vi "Get Test Configuration Properties.vi"(8 "error in (no error)":errorcluster, 11 "Routing and Faulting System Tests in":refnum<class "Routing and Faulting System Tests.lvclass">) -> (0 "error out":errorcluster, 3 "Routing and Faulting System Tests out":refnum<class "Routing and Faulting System Tests.lvclass">)   [LabVIEW 2017, in "Routing and Faulting System Tests.lvclass"]
uses:
  Routing and Faulting System Tests.lvclass
  C:/dev/CustomDevice/niveristand-custom-device-testing-tools/VeriStandTestCase/VeriStandTestCase.lvclass
  Routing and Faulting System Tests.lvclass/Routing and Faulting System Tests.ctl
  niveristand-custom-device-testing-tools/VeriStandTestCase/VeriStandTestCase.lvclass
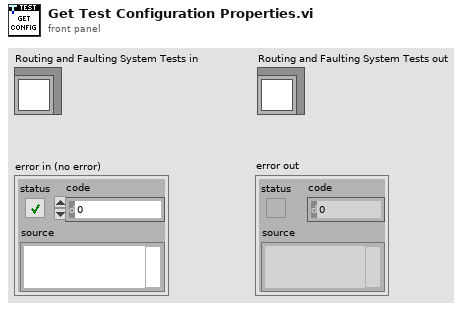
[diagram p1: front panel]
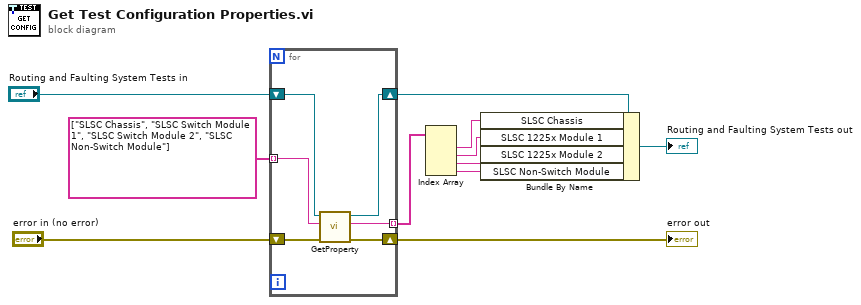
[diagram p0: block diagram]
diagram:
  n1 = for {
    tunnel: [w16] -> w6 mode=indexing
    shift-right: [w13] -> w3
    shift-left: "error in (no error)" -> [w15]
    tunnel: string[] ["SLSC Chassis", "SLSC Switch Module 1", "SLSC Switch Module 2", "SLSC Non-Switch Module"] -> [w14] mode=indexing
    shift-right: [w12] -> w1
    shift-left: "Routing and Faulting System Tests in" -> [w17]
    n2 = call "GetProperty.vi"("error in (no error)"=w15, "key"=w14, "VeriStandTestCase in"=w17) -> ("error out"=w13:errorcluster, "value"=w16:string, "VeriStandTestCase out"=w12:refnum<class "Routing and Faulting System Tests.lvclass">)  [unwired: 6 in]
  }
  "error out" <- w3
  n3 = Index Array(array=w6) -> (element #1=w7:string, element #2=w8:string, element #3=w9:string, element #4=w10:string)  [unwired: 4 in]
  n4 = Bundle By Name(cluster=w1, "SLSC Chassis"=w7, "SLSC 1225x Module 1"=w8, "SLSC 1225x Module 2"=w9, "SLSC Non-Switch Module"=w10) -> (→"Routing and Faulting System Tests out":refnum<class "Routing and Faulting System Tests.lvclass">)
